vi "Start Drag.vi"(8 "error in (no error)":errorcluster, 9 "Drag Mode":enum32{"copy or move", "copy only", "move only"}(ring), 10 "Drag Data":T1(array[cluster]), 11 "Control in":refnum<class "Control.lvclass">) -> (0 "error out":errorcluster, 3 "Control out":refnum<class "Control.lvclass">)   [LabVIEW 2015, in "Control.lvclass"]
doc: "Starts a drag and drop operation using the specified control as the source.\n\n You can use this method to start drag and drop operations in response to user-defined actions instead of the built-in behavior with string, tree, listbox, and multicolumn listbox controls. For controls other than the string, tree, listbox, and multicolumn listbox, the Start Drag method is the only way to start a drag using this control as a drag source. \n\n\nYou must specify what data to provide during the drag and drop operation. Optionally, you can specify the drag mode, and corresponding default cursor feedback, to reflect whether this drag and drop operation supports moving the data instead of only copying it. During a drag and drop operation, only drag and drop events are available. Mouse events are not available.\n\n\nIf there is already a drag in progress, LabVIEW returns an error. If you pass an empty array for the data parameter, the drag operation does not start and LabVIEW returns an error. If the array of data passed contains duplicate data names or data that conflicts with built-in types, LabVIEW returns an error.\n\n\nAfter you use this method, LabVIEW remains in the middle of a drag and drop operation until the user cancels the drag by pressing the key or lifting the mouse button, or until a window opens in front of the window that has the source control.\n\n\nThe <b>Drag Data</b> parameter is an array of clusters, each cluster containing a label and corresponding data. Each label must be unique and cannot use the LV_ prefix. Each element of the array must be of the same data type. The <b>Drag Mode</b> parameter specifies the operation of the drag, such as copy, move, or copy and move. If you select copy or move, pressing the &#60;Ctrl&#62; key copies the item.\n\n Example\n\nQControl Class wrapper around the <b>Control : Start Drag Method</b>.\n<b> </b> <b> </b>\n©2016 Q Software Innovations, LLC (QSI)\nwritten by Quentin Alldredge\nproduced in LabVIEW 2015\n\nsupport@qsoftwareinnovations.com\nwww.qsoftwareinnovations.com\n\nAll rights reserved.\n\nRedistribution and use in source and binary forms, with or without modification, are permitted provided that the following conditions are met:\n\n * Redistributions of source code must retain the above copyright notice, this list of conditions and the following disclaimer.\n * Redistributions in binary form must reproduce the above copyright notice, this list of conditions and the following disclaimer in the documentation and/or other materials provided with the distribution.\n * Neither the name of Q Software Innovations, LLC. nor the names of its contributors may be used to endorse or promote products derived from this software without specific prior written permission.\n\nTHIS SOFTWARE IS PROVIDED BY THE COPYRIGHT HOLDERS AND CONTRIBUTORS \"AS IS\" AND ANY EXPRESS OR IMPLIED WARRANTIES, INCLUDING, BUT NOT LIMITED TO, THE IMPLIED WARRANTIES OF MERCHANTABILITY AND FITNESS FOR A PARTICULAR PURPOSE ARE DISCLAIMED. IN NO EVENT SHALL THE COPYRIGHT OWNER OR CONTRIBUTORS BE LIABLE FOR ANY DIRECT, INDIRECT, INCIDENTAL, SPECIAL, EXEMPLARY, OR CONSEQUENTIAL DAMAGES (INCLUDING, BUT NOT LIMITED TO, PROCUREMENT OF SUBSTITUTE GOODS OR SERVICES; LOSS OF USE, DATA, OR PROFITS; OR BUSINESS INTERRUPTION) HOWEVER CAUSED AND ON ANY THEORY OF LIABILITY, WHETHER IN CONTRACT, STRICT LIABILITY, OR TORT (INCLUDING NEGLIGENCE OR OTHERWISE) ARISING IN ANY WAY OUT OF THE USE OF THIS SOFTWARE, EVEN IF ADVISED OF THE POSSIBILITY OF SUCH DAMAGE."
uses:
  Control.lvclass
  Control.lvclass/Control.ctl
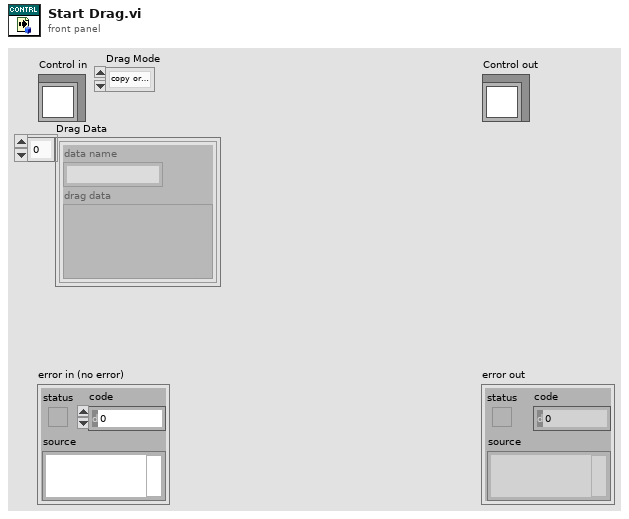
[diagram p1: front panel]
types:
  T1 = cluster{"data name":string, "drag data":variant}[]
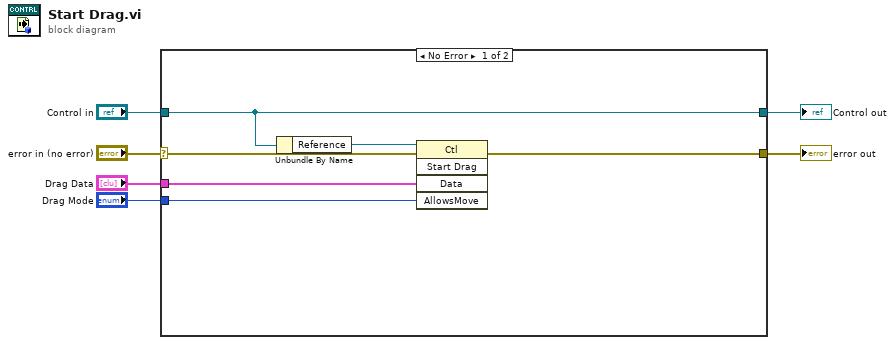
[diagram p0: block diagram]
diagram:
  n1 = case shown="No Error" "error in (no error)" {
    selector: "error in (no error)" -> [w12 w14]
    tunnel: [w11 w14] -> w5
    tunnel: [w10 w13] -> w3
    tunnel: "Control in" -> [w10 w13]
    tunnel: "Drag Data" -> [w8 _]
    tunnel: "Drag Mode" -> [w7 _]
    frame No Error {
      n2 = Unbundle By Name(w10) -> ("Reference"=w9:refnum<vi>)
      n3 = invoke class="Ctl" method="Start Drag"(reference=w9, error in=w12, "Data"=w8, "AllowsMove"=w7) -> (error out=w11:errorcluster)  [unwired: 1 in, 4 out]
    }
    frame Error {
    }
  }
  "error out" <- w5
  "Control out" <- w3
